vi "to string.vi"(8 "error in":errorcluster, 11 "Sync Channel configuration in":refnum<class "Synchronization Channel configuration.lvclass">) -> (0 "error out":errorcluster, 1 "data":string, 2 "version":string, 3 "Sync Channel configuration out":refnum<class "Synchronization Channel configuration.lvclass">)   [LabVIEW 2025, in "Synchronization.lvlib" / "Synchronization Channel configuration.lvclass"]
doc: "Provides an interface for saving a module configuration to a file or other serialized data source. It is recommended that all children of this class store data in two sets--data required for its own initialization, and any data required for parent initialization--and that each implementation uses the <b>Call Parent Method</b> primitive to serialize parent information.Copyright 2017 National Instruments Corporation\n\nLicensed under the Apache License, Version 2.0 (the \"License\"); you may not use this file except in compliance with the License. You may obtain a copy of the License at http://www.apache.org/licenses/LICENSE-2.0\nUnless required by applicable law or agreed to in writing, software distributed under the License is distributed on an \"AS IS\" BASIS, WITHOUT WARRANTIES OR CONDITIONS OF ANY KIND, either express or implied. See the License for the specific language governing permissions and limitations under the License."
uses:
  Synchronization Channel configuration.lvclass
  Synchronization Channel configuration.lvclass/Synchronization Channel configuration.ctl
  Users/Public/Documents/Sandia National Labs/TSS Plugin/Abstract Engine.lvlibp/Plugin/Abstract/Channel configuration/Channel configuration.lvclass
  Users/Public/Documents/Sandia National Labs/TSS Plugin/CEF.lvlibp/serializable configuration/CEF_serializable configuration.lvclass
  Users/Public/Documents/Sandia National Labs/TSS Plugin/CEF.lvlibp
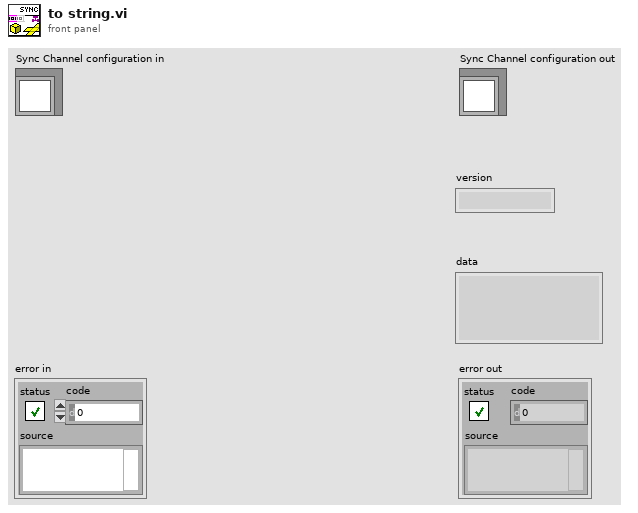
[diagram p1: front panel]
types:
  T1 = typedef "Synchronization.lvlib/Synchronization Channel configuration.lvclass/Sync Channel Setting.ctl" = cluster{"Inverter":bool, "Update Edge":string, "Source":string, "Type":string, "Synchronization Clock":string, "Destination":string}
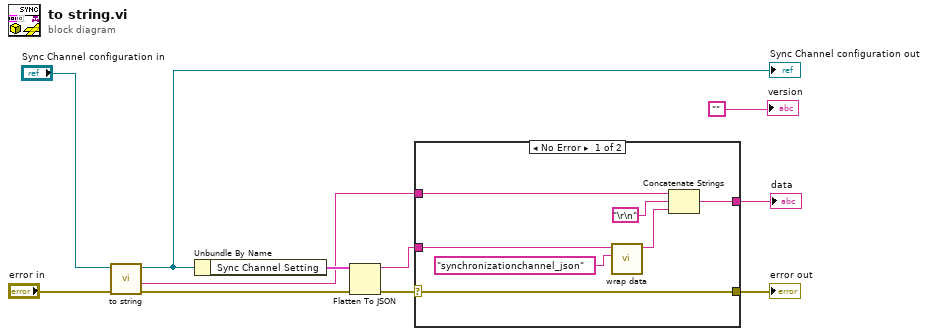
[diagram p0: block diagram]
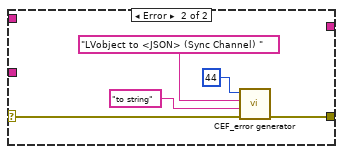
[diagram p2: hidden frame]
diagram:
  n1 = call-parent "to string.vi"("error in"="error in", "Channel configuration"="Sync Channel configuration in") -> ("error out"=w8:errorcluster, "data"=w3:string, "Channel configuration out"=w9:refnum<class "Synchronization Channel configuration.lvclass">)  [unwired: 6 in, 1 out]
  "Sync Channel configuration out" <- w9
  n2 = Unbundle By Name(w9) -> ("Sync Channel Setting"=w7:T1)
  n3 = Flatten To JSON(anything=w7, error in (no error)=w8) -> (JSON string=w4:string, 11:w6:errorcluster)  [unwired: 1 in]
  n4 = case shown="No Error" w6 {
    selector: w6 -> [w18 w20]
    tunnel: [w18 w19] -> w5
    tunnel: w4 -> [w15 _]
    tunnel: w3 -> [w14 _]
    tunnel: [w12 _] -> w2
    frame No Error {
      n5 = call "wrap data.vi"("identifier"="synchronizationchannel_json" ("additional identifier"), "data to wrap"=w15) -> ("wrapped data"=w17:string)  [unwired: 9 in]
      n6 = Concatenate Strings(w14, "\r\n", w17) -> (w12:string)
    }
    frame Error {
      n7 = call "CEF_error generator.vi"("error in"=w20, "source"="to string" ("message"), "append error message"="LVobject to <JSON> (Sync Channel) " ("message"), "error code (0)"=44) -> ("error out"=w19:errorcluster)  [unwired: 5 in]
    }
  }
  "error out" <- w5
  "data" <- w2
  "version" <- ""
